vi "Transform error.vi"(8 "error in (no error)":errorcluster, 9 "server errors":u8[](array[numeric]), 10 "return code":u8, 11 "client in":refnum<class "OpenSSH Client.lvclass">) -> (0 "error out":errorcluster, 1 "server errors out":u8[](array[numeric]), 2 "return code out":u8, 3 "client out":refnum<class "OpenSSH Client.lvclass">)   [LabVIEW 2020, in "NI_SSH.lvlib" / "OpenSSH Client.lvclass"]
uses:
  <vilib>/net/SSH/Client/OpenSSH/OpenSSH Client.lvclass
  <vilib>/net/SSH/Client/Generic/Stderr Match Patterns.ctl
  <vilib>/net/SSH/Client/Generic/Generic Client.lvclass
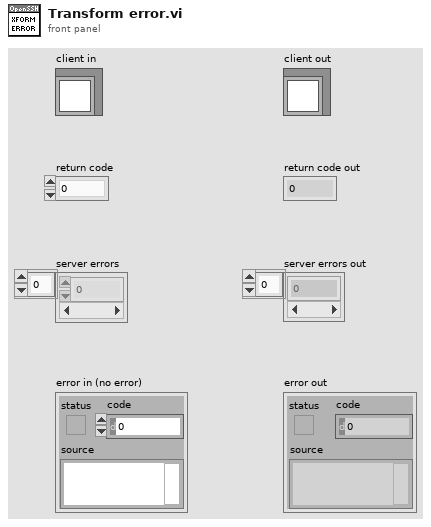
[diagram p1: front panel]
types:
  T1 = typedef "NI_SSH.lvlib/Generic Client.lvclass/Stderr Match Patterns.ctl" = cluster{"incorrect pubkey":string, "unknown pubkey":string, "crypto disallowed":string, "dns spoofing":string, "access denied":string}
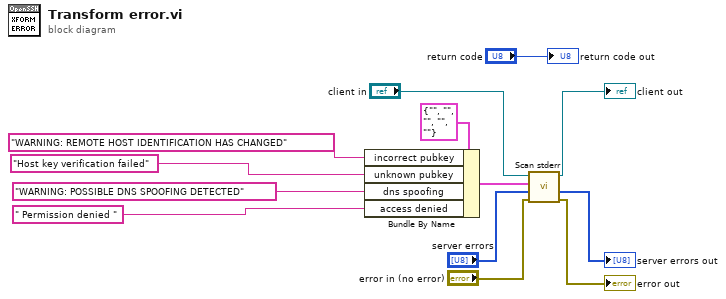
[diagram p0: block diagram]
diagram:
  n1 = Bundle By Name(cluster=T1 {"incorrect pubkey"="", "unknown pubkey"="", "crypto disallowed"="", "dns spoofing"="", "access denied"=""} ("patterns"), "incorrect pubkey"="WARNING: REMOTE HOST IDENTIFICATION HAS CHANGED" ("regular expression"), "unknown pubkey"="Host key verification failed" ("regular expression"), "dns spoofing"="WARNING: POSSIBLE DNS SPOOFING DETECTED", "access denied"=" Permission denied ") -> (w10:T1)
  n2 = call-dynamic "Scan stderr.vi"("error in (no error)"="error in (no error)", "stderr in"="server errors", "patterns"=w10, "client in"="client in") -> ("error out"=→"error out":errorcluster, "stderr out"=→"server errors out":u8[], "client out"=→"client out":refnum<class "OpenSSH Client.lvclass">)  [unwired: 5 in]
  "return code out" <- "return code"
